vi "HEWH Standard Ambient Checker.vi"(7 "Water Heater Type":T1, 10 "Heat Source_Array":u8[](array[numeric]), 11 "Ambient_Temp_Array":dbl[](array[numeric])) -> (1 "Ambient Temp (Full Range)":bool, 2 "Ambient Temperature Min Value":dbl, 3 "Ambient Temperature Max Value":dbl)   [LabVIEW 2023]
uses:
  Type Definitions/HEWH Water Heater Type.ctl
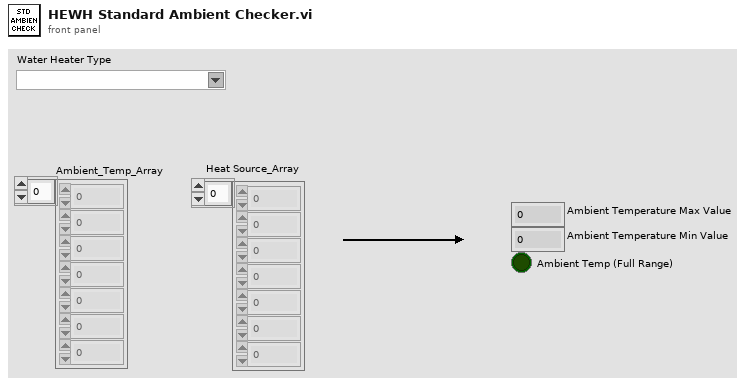
[diagram p1: front panel]
types:
  T1 = typedef "HEWH Water Heater Type.ctl" = string
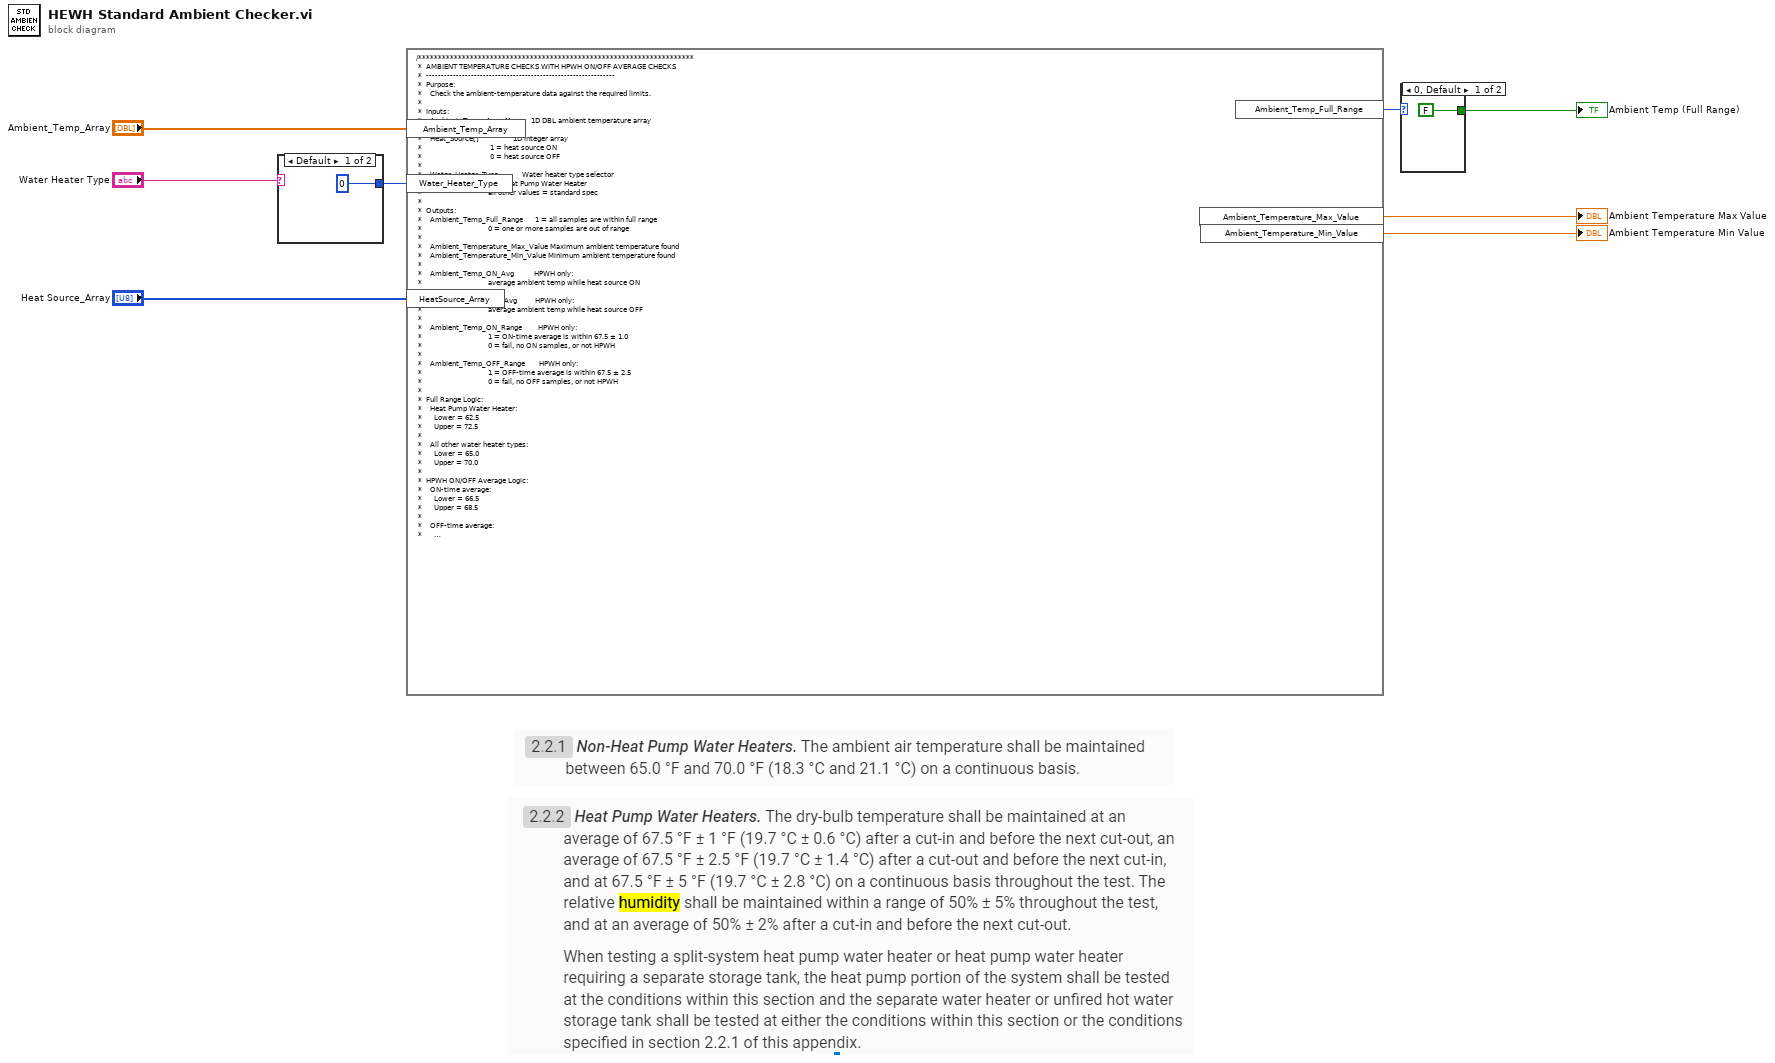
[diagram p0: block diagram]
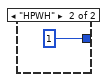
[diagram p2: hidden frame]
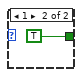
[diagram p3: hidden frame]
diagram:
  n1 = case shown="Default" "Water Heater Type" {
    tunnel: [0 ("Water_Heater_Type") 1 ("Water_Heater_Type")] -> w2
    frame Default {
    }
    frame "HPWH" {
    }
  }
  n2 = formula code="/*********************************************************************\n *  AMBIENT TEMPERATURE CHECKS WITH HPWH ON/OFF AVERAGE CHECKS\n *  ---------------------------------------------------------------\n *  Purpose:\n *    Check the ambient-temperature data against the required limits.\n *\n *  Inputs:\n *    Ambient_Temp_Array[]          1D DBL ambient temperature array\n *\n *    Heat_Source[]                 1D integer array\n *                                  1 = heat source ON\n *                                  0 = heat source OFF\n *\n *    Water_Heater_Type            Water heater type selector\n *                                 1 = Heat Pump Water Heater\n *                                 all other values = standard spec\n *\n *  Outputs:\n *    Ambient_Temp_Full_Range      1 = all samples are within full range\n *                                 0 = one or more samples are out of range\n *\n *    Ambient_Temperature_Max_Value Maximum ambient temperature found\n *    Ambient_Temperature_Min_Value Minimum ambient temperature found\n *\n *    Ambient_Temp_ON_Avg          HPWH only:\n *                                 average ambient temp while heat source ON\n *\n *    Ambient_Temp_OFF_Avg         HPWH only:\n *                                 average ambient temp while heat source OFF\n *\n *    Ambient_Temp_ON_Range        HPWH only:\n *                                 1 = ON-time average is within 67.5 ± 1.0\n *                                 0 = fail, no ON samples, or not HPWH\n *\n *    Ambient_Temp_OFF_Range       HPWH only:\n *                                 1 = OFF-time average is within 67.5 ± 2.5\n *                                 0 = fail, no OFF samples, or not HPWH\n *\n *  Full Range Logic:\n *    Heat Pump Water Heater:\n *      Lower = 62.5\n *      Upper = 72.5\n *\n *    All other water heater types:\n *      Lower = 65.0\n *      Upper = 70.0\n *\n *  HPWH ON/OFF Average Logic:\n *    ON-time average:\n *      Lower = 66.5\n *      Upper = 68.5\n *\n *    OFF-time average:\n *      Lower = 65.0\n *      Upper = 70.0\n *********************************************************************/\n\n\n/* ---------------- Local variables -------------------------------- */\n\nint32 i;\nint32 N;\nint32 N_Heat;\nint32 Loop_N;\n\nint32 ON_Count;\nint32 OFF_Count;\n\nfloat Selected_Upper_Spec;\nfloat Selected_Lower_Spec;\n\nfloat ON_Upper_Spec;\nfloat ON_Lower_Spec;\n\nfloat OFF_Upper_Spec;\nfloat OFF_Lower_Spec;\n\nfloat Ambient_Value;\nfloat ON_Sum;\nfloat OFF_Sum;\n\n\n/* ---------------- Default outputs -------------------------------- */\n\nint32 Ambient_Temp_Full_Range = 0;\n\nAmbient_Temperature_Max_Value = 0.0;\nAmbient_Temperature_Min_Value = 0.0;\n\nAmbient_Temp_ON_Avg = 0.0;\nAmbient_Temp_OFF_Avg = 0.0;\n\nAmbient_Temp_ON_Range = 0;\nAmbient_Temp_OFF_Range = 0;\n\n\n/* ---------------- Default local values ---------------------------- */\n\nON_Count = 0;\nOFF_Count = 0;\n\nON_Sum = 0.0;\nOFF_Sum = 0.0;\n\n\n/* ---------------- Select full-range specification ----------------- */\n\nif (Water_Heater_Type == 1)\n{\n    /*\n     * Heat Pump Water Heater full-range ambient specification.\n     */\n\n    Selected_Upper_Spec = 67.5 + 5.0;\n    Selected_Lower_Spec = 67.5 - 5.0;\n}\nelse\n{\n    /*\n     * Standard full-range ambient specification for all other types.\n     */\n\n    Selected_Upper_Spec = 70.0;\n    Selected_Lower_Spec = 65.0;\n}\n\n\n/* ---------------- HPWH ON/OFF average specifications -------------- */\n\nON_Upper_Spec = 67.5 + 1.0;\nON_Lower_Spec = 67.5 - 1.0;\n\nOFF_Upper_Spec = 67.5 + 2.5;\nOFF_Lower_Spec = 67.5 - 2.5;\n\n\n/* ---------------- Get array lengths ------------------------------- */\n\nN = sizeOfDim(Ambient_Temp_Array, 0);\nN_Heat = sizeOfDim(Heat_Source, 0);\n\n\n/* ---------------- Evaluate ambient temperature data --------------- */\n\nif (N > 0)\n{\n    /*\n     * Initialize min and max using the first sample.\n     */\n\n    Ambient_Temperature_Max_Value = Ambient_Temp_Array[0];\n    Ambient_Temperature_Min_Value = Ambient_Temp_Array[0];\n\n\n    /*\n     * Loop through the remaining array values and find the maximum\n     * and minimum ambient temperature values.\n     */\n\n    for (i = 1; i < N; i++)\n    {\n        Ambient_Value = Ambient_Temp_Array[i];\n\n\n        if (Ambient_Value > Ambient_Temperature_Max_Value)\n        {\n            Ambient_Temperature_Max_Value = Ambient_Value;\n        }\n\n\n        if (Ambient_Value < Ambient_Temperature_Min_Value)\n        {\n            Ambient_Temperature_Min_Value = Ambient_Value;\n        }\n    }\n\n\n    /*\n     * Check the full data range against the selected limits.\n     * This applies to both HPWH and non-HPWH units.\n     */\n\n    if (Ambient_Temperature_Max_Value <= Selected_Upper_Spec &&\n        Ambient_Temperature_Min_Value >= Selected_Lower_Spec)\n    {\n        Ambient_Temp_Full_Range = 1;\n    }\n    else\n    {\n        Ambient_Temp_Full_Range = 0;\n    }\n\n\n    /*****************************************************************\n     * HPWH ONLY:\n     *   Check average ambient temperature while heat source is ON\n     *   and while heat source is OFF.\n     *****************************************************************/\n\n    if (Water_Heater_Type == 1)\n    {\n        /*\n         * Only run ON/OFF checks if the Heat_Source array has data.\n         */\n\n        if (N_Heat > 0)\n        {\n            /*\n             * Use the smaller array length if Ambient_Temp_Array and\n             * Heat_Source are not the same size.\n             */\n\n            Loop_N = N;\n\n            if (N_Heat < Loop_N)\n            {\n                Loop_N = N_Heat;\n            }\n\n\n            /*\n             * Separate ambient samples into ON-time and OFF-time groups.\n             */\n\n            for (i = 0; i < Loop_N; i++)\n            {\n                if (Heat_Source[i] == 1)\n                {\n                    ON_Sum += Ambient_Temp_Array[i];\n                    ON_Count += 1;\n                }\n                else if (Heat_Source[i] == 0)\n                {\n                    OFF_Sum += Ambient_Temp_Array[i];\n                    OFF_Count += 1;\n                }\n            }\n\n\n            /*\n             * Calculate ON-time average and check tolerance.\n             */\n\n            if (ON_Count > 0)\n            {\n                Ambient_Temp_ON_Avg = ON_Sum / ON_Count;\n\n                if (Ambient_Temp_ON_Avg >= ON_Lower_Spec &&\n                    Ambient_Temp_ON_Avg <= ON_Upper_Spec)\n                {\n                    Ambient_Temp_ON_Range = 1;\n                }\n                else\n                {\n                    Ambient_Temp_ON_Range = 0;\n                }\n            }\n            else\n            {\n                Ambient_Temp_ON_Avg = 0.0;\n                Ambient_Temp_ON_Range = 0;\n            }\n\n\n            /*\n             * Calculate OFF-time average and check tolerance.\n             */\n\n            if (OFF_Count > 0)\n            {\n                Ambient_Temp_OFF_Avg = OFF_Sum / OFF_Count;\n\n                if (Ambient_Temp_OFF_Avg >= OFF_Lower_Spec &&\n                    Ambient_Temp_OFF_Avg <= OFF_Upper_Spec)\n                {\n                    Ambient_Temp_OFF_Range = 1;\n                }\n                else\n                {\n                    Ambient_Temp_OFF_Range = 0;\n                }\n            }\n            else\n            {\n                Ambient_Temp_OFF_Avg = 0.0;\n                Ambient_Temp_OFF_Range = 0;\n            }\n        }\n    }\n}\nelse\n{\n    /*\n     * Empty ambient array fault.\n     */\n\n    Ambient_Temp_Full_Range = 0;\n\n    Ambient_Temperature_Max_Value = 0.0;\n    Ambient_Temperature_Min_Value = 0.0;\n\n    Ambient_Temp_ON_Avg = 0.0;\n    Ambient_Temp_OFF_Avg = 0.0;\n\n    Ambient_Temp_ON_Range = 0;\n    Ambient_Temp_OFF_Range = 0;\n}"("Ambient_Temp_Array"="Ambient_Temp_Array", "Water_Heater_Type"=w2, "HeatSource_Array"="Heat Source_Array") -> ("Ambient_Temp_Full_Range"=w5:i32, "Ambient_Temperature_Max_Value"=→"Ambient Temperature Max Value":dbl, "Ambient_Temperature_Min_Value"=→"Ambient Temperature Min Value":dbl)
  n3 = case shown="0, Default" w5 {
    tunnel: [FALSE TRUE] -> w4
    frame 0, Default {
    }
    frame 1 {
    }
  }
  "Ambient Temp (Full Range)" <- w4
